vi "set_currents.vi"(10 "Device Handle Out":u32, 11 "REACTORS":T1(array[cluster])) -> (2 "Device Handle Out 2":u32, 3 "REACTORS 2":T1(array[cluster]))   [LabVIEW 2013]
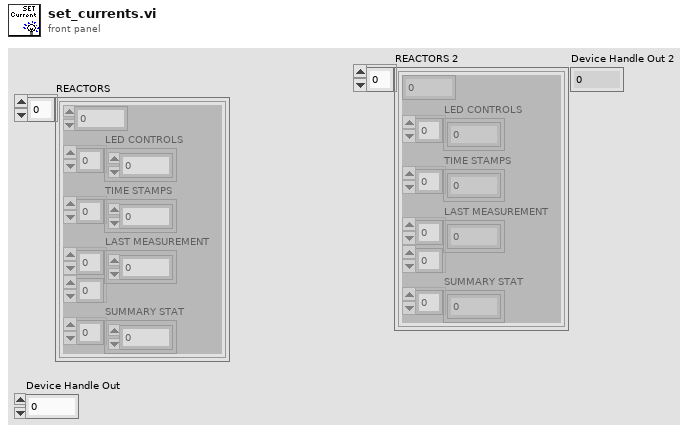
[diagram p1: front panel]
types:
  T1 = cluster{i32, "LED CONTROLS":dbl[], "TIME STAMPS":dbl[], "LAST MEASUREMENT":dbl[][], "SUMMARY STAT":dbl[]}[]
  T2 = enum16{"Set Mode", "Set Normal Current ", "Set Strobe Parameters", "Set Normal Parameters", "Set Strobe Profile "}
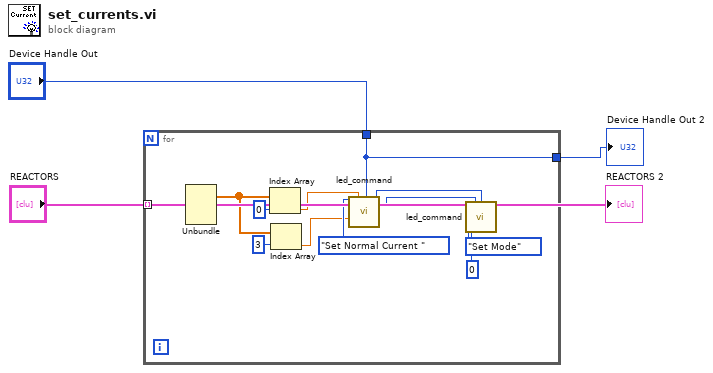
[diagram p0: block diagram]
diagram:
  n1 = for {
    tunnel: "REACTORS" -> [w14] mode=indexing
    tunnel: "Device Handle Out" -> [w4]
    tunnel: [w4] -> w1
    n2 = Unbundle(w14) -> ("LED CONTROLS"=w10:dbl[])  [unwired: 4 out]
    n3 = Index Array(array=w10, index=0) -> (element=w12:dbl)
    n4 = Index Array(array=w10, index=3) -> (element=w9:dbl)
    n5 = call "led_command.vi"("COMMAND"=T2."Set Normal Current ", "Channel"=w12, "Device Handle"=w4, "Iset"=w9) -> ("Device Handle Out"=w6:u32, "Channel Out"=w7:i32)  [unwired: 8 in, 2 out]
    n6 = call "led_command.vi"("COMMAND"=T2."Set Mode", "Channel"=w7, "Device Handle"=w6, "Mode"=u32 0) -> ()  [unwired: 8 in, 4 out]
  }
  "Device Handle Out 2" <- w1
  "REACTORS 2" <- "REACTORS"
